vi "TrianglePattern.vi"(5 "Phase (2pi unit)":dbl, 9 "Ratio":dbl=20.0, 11 "N":i32) -> (1 "vector":dbl[](array[numeric]), 3 "points":i32[](array[numeric]))   [LabVIEW 2015, in "ArbitraryFunctions.lvlib"]
uses:
  ArbitraryFunctions.lvlib
panel:
  out "Waveform OUT":dbl[](graph)
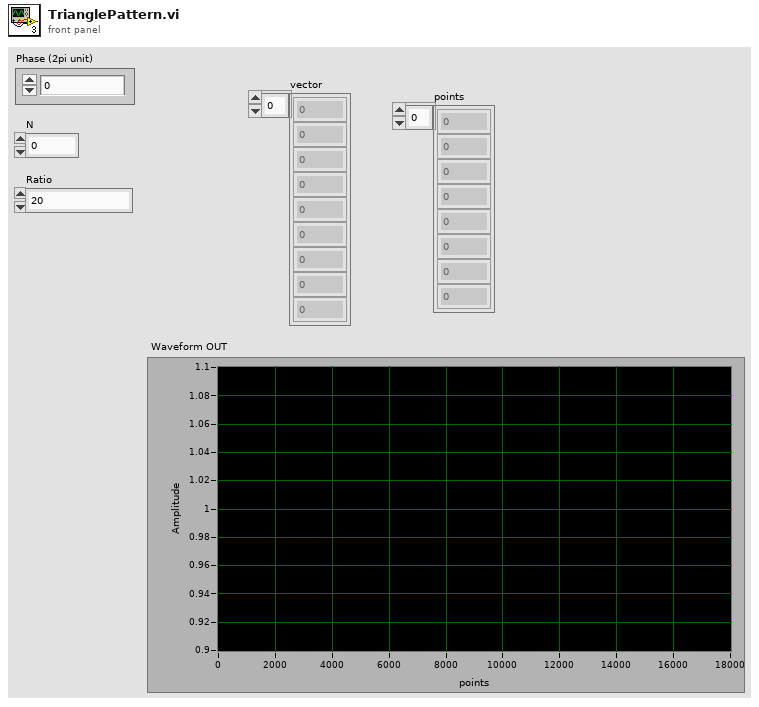
[diagram p1: front panel]
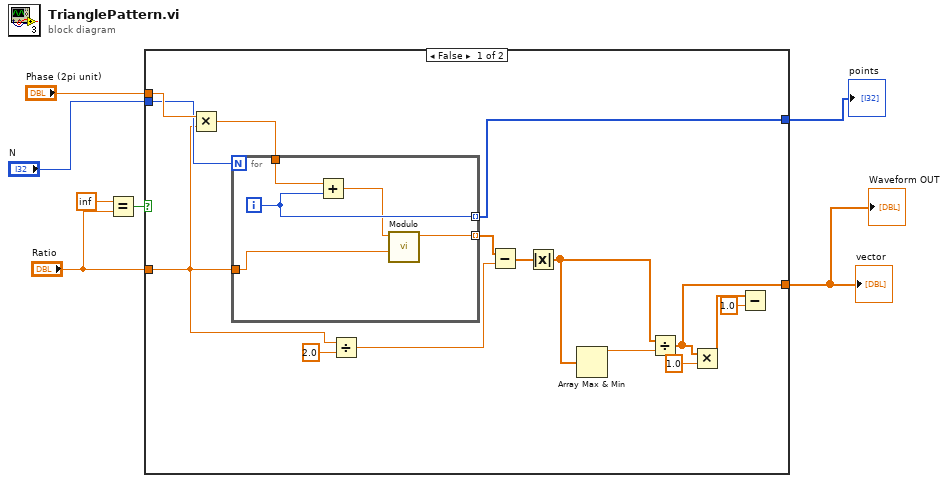
[diagram p0: block diagram]
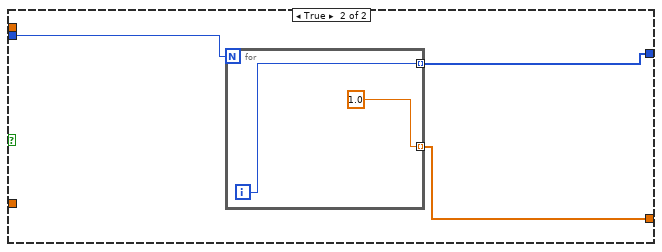
[diagram p2: hidden frame]
diagram:
  n1 = Equal?(x=inf, y="Ratio") -> (x = y?=w1:bool)
  n2 = case shown="False" w1 {
    tunnel: "Phase (2pi unit)" -> [w15 _]
    tunnel: "N" -> [w13 w30]
    tunnel: [w10 w29] -> w5
    tunnel: "Ratio" -> [w8 _]
    tunnel: [w9 w28] -> w4
    frame False {
      n3 = Multiply(x=w15, y=w8) -> (x*y=w16:dbl)
      n4 = for {
        N: w13 -> [_]
        tunnel: [w25] -> w9 mode=indexing
        tunnel: [w26] -> w12 mode=indexing
        tunnel: w8 -> [w27]
        tunnel: w16 -> [w24]
        i -> [w25]
        n5 = Add(x=w24, y=w25) -> (x+y=w23:dbl)
        n6 = call "Modulo.vi"("mod"=w27, "input"=w23) -> ("output"=w26:dbl)  [unwired: 8 in, 1 out]
      }
      n7 = Divide(x=w8, y=2.0) -> (x/y=w17:dbl)
      n8 = Subtract(x=w12, y=w17) -> (x-y=w11:dbl[])
      n9 = Absolute Value(x=w11) -> (abs(x)=w14:dbl[])
      n10 = Array Max & Min(array=w14) -> (max value=w19:dbl)  [unwired: 3 out]
      n11 = Divide(x=w14, y=w19) -> (x/y=w10:dbl[])
      n12 = Multiply(x=w10, y=1.0) -> (x*y=w20:dbl[])
      n13 = Subtract(x=w20, y=1.0) -> ()  [unwired: 1 out]
    }
    frame True {
      n14 = for {
        N: w30 -> [_]
        tunnel: [1.0 ("output")] -> w29 mode=indexing
        tunnel: [w31] -> w28 mode=indexing
        i -> [w31]
      }
    }
  }
  "vector" <- w5
  "Waveform OUT" <- w5
  "points" <- w4
